vi "FPGA_Check_Pins_host.vi"() -> ()   [LabVIEW 2018]
uses:
  <vilib>/userdefined/High Color/nirio_resource_hc.ctl
  <vilib>/FPGAPlugInAG/PXI-7951R/niLvFpga_Open_PXI-7951R.vi
  <vilib>/rvi/interface/common/dynamic/niFpgaDynamicAddResources.vi
  <vilib>/FPGAPlugInAG/Dynamic/niLvFpga_Reset_Dynamic.vi
  <vilib>/FPGAPlugInAG/Dynamic/niLvFpga_Run_Dynamic.vi
  <vilib>/Utility/error.llb/Error Cluster From Error Code.vi
  <vilib>/rvi/errors/niLvFpgaAdjustHostInterfaceError.vi
  <vilib>/FPGAPlugInAG/Dynamic/niLvFpga_Close_Dynamic.vi
  <vilib>/rvi/interface/nirviOpenFPGA/nirviOpenFPGA.xnode
  FPGA Bitfiles/FPGACheckPins_FPGATarget_FPGACheckPinstar_o4gGUkoAHio.lvbitx
  <vilib>/rvi/interface/nirviMethod/nirviMethod.xnode
  <vilib>/rvi/interface/nirviReadWriteControl/nirviReadWriteControl.xnode
  <vilib>/rvi/interface/nirviCloseFPGA/nirviCloseFPGA.xnode
  <vilib>/rvi/interface/Simulation/niFpgaSimulationCallBeginRW.vi
  NiFpgaLv.dll
panel:
  in  "Tab Control":enum32{"Main", "Service"}(tab)
  out "output array":bool[][](array[boolean])
  out "appended array":bool[](array[boolean])
  out "Ток, А":dbl(knob) scale=0.0..1.0
  in  "FPGA slot name":T1="PXI1Slot2" caption="RIO Device"
  out "error out (4110)":errorcluster
  out "error out FPGA":errorcluster
  in  "Power Resource":refnum<k15>="PXI1Slot3"
  in  "Output enabled CH1":bool
  in  "Stop Program":bool
  in  "Write to Read":bool
  out "Read B":u32=117440511 format="%b"
  out "Read A":u32=134217727 format="%b"
  out "WRITE TOTAL":u32=38686286 format="%b"
  in  "Ток, А  2":dbl=0.9 caption="Current limit CH1" format="%#_13g"
  in  "Напряжение, В":dbl=3.0
  out "U CH0.1, В":dbl=0.000596728952024882
  out "I CH0.1, A":dbl=2.324707150327661e-06
  in  "Write to PFI 2":u8=6 format="%b"
  in  "Write to PFI":u16(ring)=1 items=["Manual mode", "Random", "Increment", "Chess", "NChess", "Only one", "Zero", "Check one"]
  in  "Cycle":bool=TRUE
  in  "Write to port  2":u8=248 format="%b"
  out "Read PFI 2":i16=1
  out "Read PFI 3":i16=1
  out "Read PFI 1":i16
  out "Чтение PFI 1":i16=1
  out "Чтение PFI 2":i16=1
  out "Чтение PFI 3":i16=1
  out "Read B2":u32=255 format="%b"
  out "Read B1":u32=255 format="%b"
  out "Read B0":u32=255
  out "Read А2":u32=255 format="%b"
  out "Read А1":u32=255 format="%b"
  out "Read А0":u32=255
  in  "Write to port":u16(ring)=1 items=["Manual mode", "Random", "Increment", "Chess", "NChess", "Only one", "Zero", "Chess diagonal", "NChess diagonal"]
  out "Delay B to A, такт":i16
  out "Delay A to B, такт":i16
  # "0          1          2         3          4          5          6          7"
  # "Port 0"
  # "PFI 1"
  # "Port 1"
  # "PFI 2"
  # "Port 2"
  # "PFI 3"
  # "Control"
  # "Чтение портов"
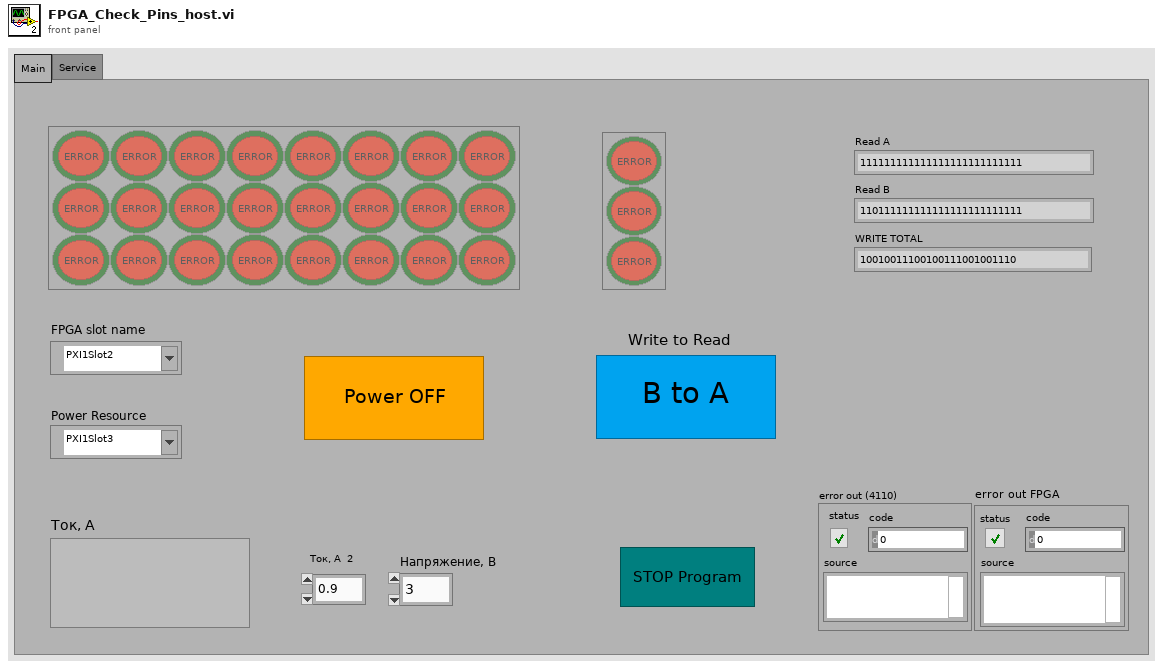
[diagram p1: front panel]
types:
  T1 = typedef "nirio_resource_hc.ctl" = tag
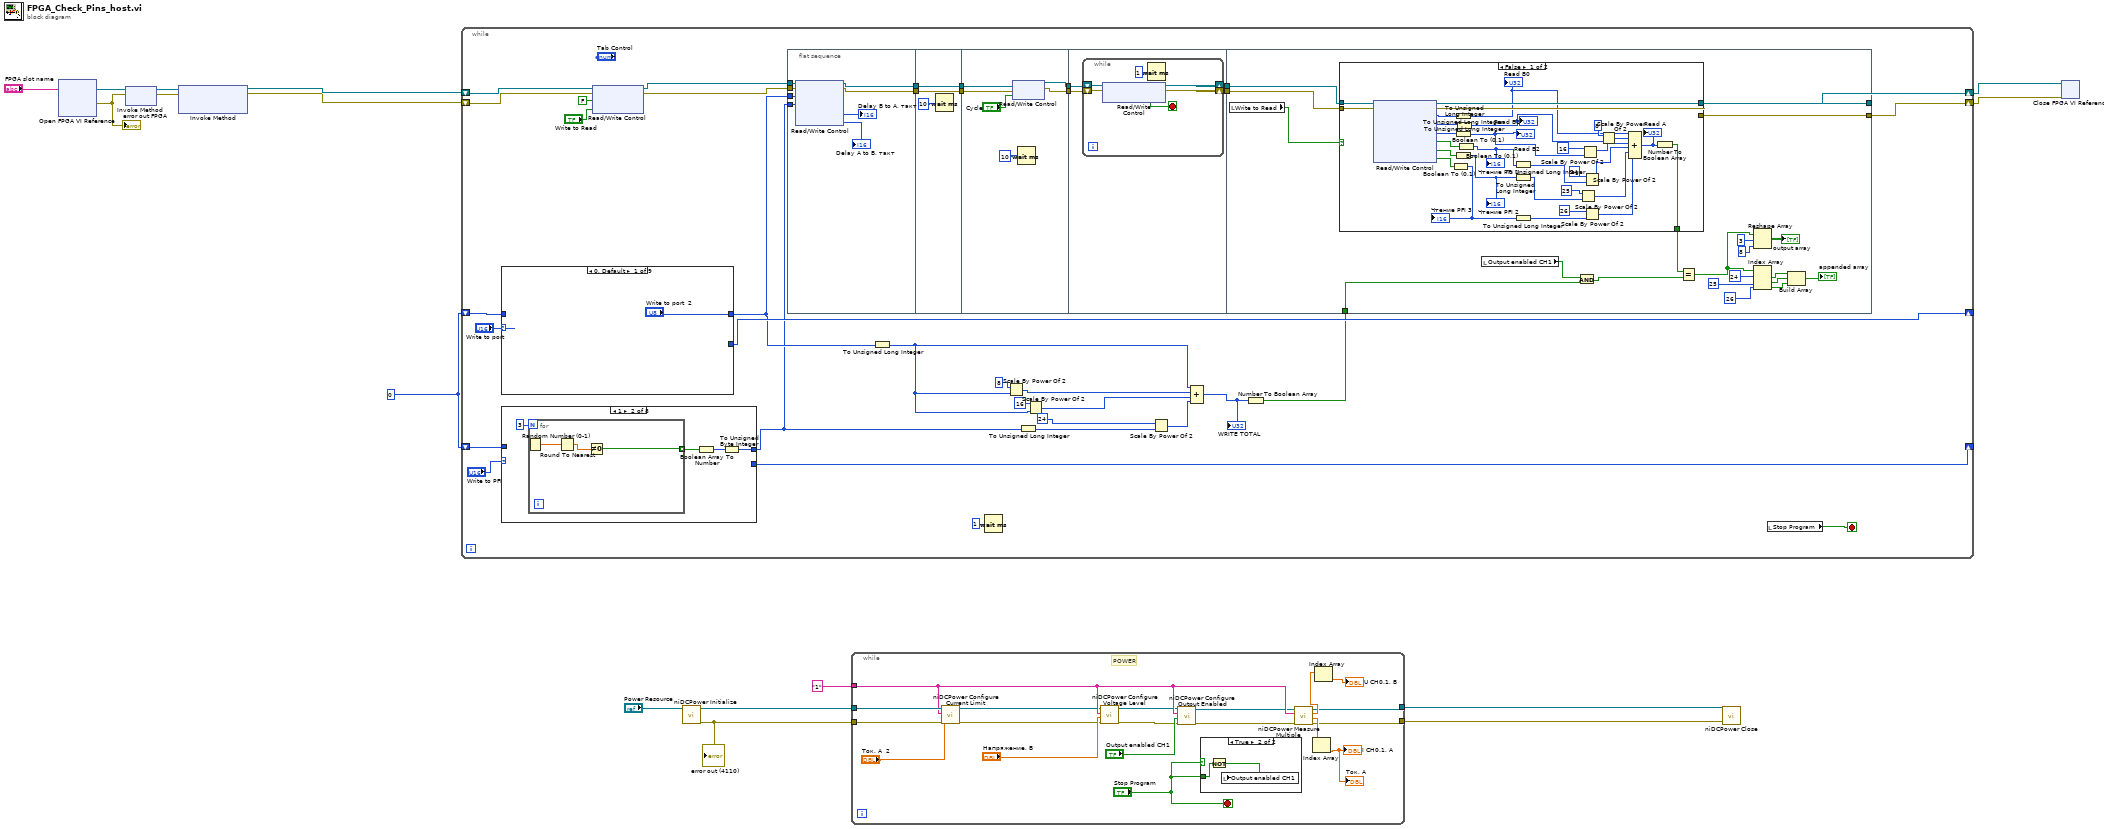
[diagram p0: block diagram]
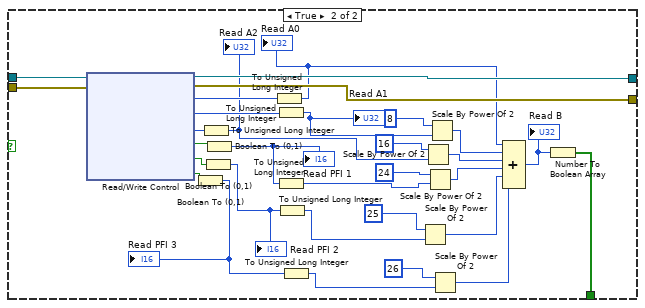
[diagram p2: hidden frame]
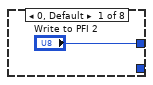
[diagram p3: hidden frame]
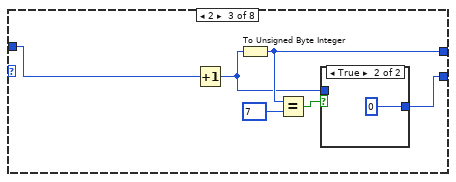
[diagram p4: hidden frame]
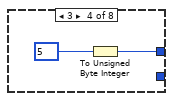
[diagram p6: hidden frame]
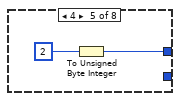
[diagram p7: hidden frame]
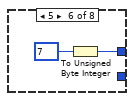
[diagram p8: hidden frame]
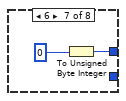
[diagram p9: hidden frame]
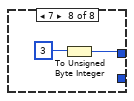
[diagram p10: hidden frame]
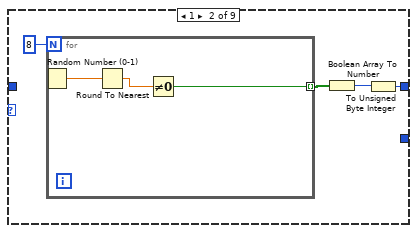
[diagram p11: hidden frame]
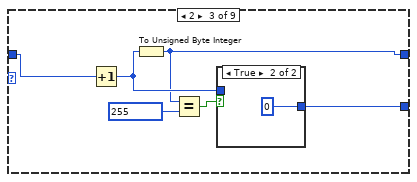
[diagram p12: hidden frame]
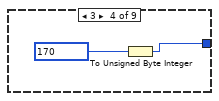
[diagram p14: hidden frame]
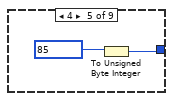
[diagram p15: hidden frame]
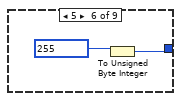
[diagram p16: hidden frame]
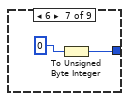
[diagram p17: hidden frame]
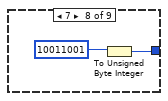
[diagram p18: hidden frame]
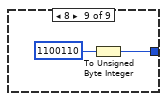
[diagram p19: hidden frame]
diagram:
  w1 = 0
  n1 = xnode "Open FPGA VI Reference"("resource name"="FPGA slot name") -> ("FPGA VI Reference Out"=w9:refnum<k20>, "error out"=w8:errorcluster)  [unwired: 1 in]
  "error out FPGA" <- w8
  n2 = xnode "Invoke Method"("FPGA VI Reference In"=w9, "error in"=w8) -> ("FPGA VI Reference Out"=w7:refnum<k20>, "error out"=w6:errorcluster)
  n3 = xnode ("Invoke Method")("FPGA VI Reference In"=w7, "error in"=w6) -> ("FPGA VI Reference Out"=w3:refnum<k20>, "error out"=w2:errorcluster)  [unwired: 1 in]
  n4 = while {
    shift-right: [w19] -> w5
    shift-left: w3 -> [w37]
    shift-right: [w18] -> w4
    shift-left: w2 -> [w36]
    shift-right: [w40] -> _
    shift-left: w1 -> [w41]
    shift-right: [w38] -> _
    shift-left: w1 -> [w39]
    stop <- w22 stop-if-true
    n5 = case shown="0, Default" "Write to port" {
      tunnel: ["Write to port  2" w189 w197 w204 w207 w209 w211 w213 w214] -> w33
      tunnel: w39 -> [_ _ w198 _ _ _ _ _ _]
      tunnel: [_ _ w196 _ _ _ _ _ _] -> w38
      frame 0, Default {
      }
      frame 1 {
        n6 = for {
          N: 8 -> [_]
          tunnel: [w193] -> w191 mode=indexing
          n7 = Random Number (0-1)() -> (number: 0 to 1=w195:dbl)
          n8 = Round To Nearest(number=w195) -> (nearest integer value=w194:dbl)
          n9 = Not Equal To 0?(x=w194) -> (x != 0?=w193:bool)
        }
        n10 = Boolean Array To Number(Boolean array=w191) -> (number=w190:u32)
        n11 = To Unsigned Byte Integer(number=w190) -> (unsigned 8bit integer=w189:u8)
      }
      frame 2 {
        n12 = Increment(x=w198) -> (x+1=w201:i32)
        n13 = To Unsigned Byte Integer(number=w201) -> (unsigned 8bit integer=w197:u8)
        n14 = Equal?(x=w197, y=u8 255) -> (x = y?=w200:bool)
        n15 = case shown="True" w200 {
          tunnel: [w202 0] -> w196
          tunnel: w201 -> [w202 _]
          frame False {
          }
          frame True {
          }
        }
      }
      frame 3 {
        n16 = To Unsigned Byte Integer(number=170) -> (unsigned 8bit integer=w204:u8)
      }
      frame 4 {
        n17 = To Unsigned Byte Integer(number=85) -> (unsigned 8bit integer=w207:u8)
      }
      frame 5 {
        n18 = To Unsigned Byte Integer(number=255) -> (unsigned 8bit integer=w209:u8)
      }
      frame 6 {
        n19 = To Unsigned Byte Integer(number=0) -> (unsigned 8bit integer=w211:u8)
      }
      frame 7 {
        n20 = To Unsigned Byte Integer(number=10011001) -> (unsigned 8bit integer=w213:u8)
      }
      frame 8 {
        n21 = To Unsigned Byte Integer(number=1100110) -> (unsigned 8bit integer=w214:u8)
      }
    }
    n22 = case shown="1" "Write to PFI" {
      tunnel: ["Write to PFI 2" w163 w173 w179 w181 w183 w185 w187] -> w30
      tunnel: w41 -> [_ _ w175 _ _ _ _ _]
      tunnel: [_ _ w171 _ _ _ _ _] -> w40
      frame 0, Default {
      }
      frame 1 {
        n23 = for {
          N: 3 -> [_]
          tunnel: [w167] -> w165 mode=indexing
          n24 = Random Number (0-1)() -> (number: 0 to 1=w169:dbl)
          n25 = Round To Nearest(number=w169) -> (nearest integer value=w168:dbl)
          n26 = Not Equal To 0?(x=w168) -> (x != 0?=w167:bool)
        }
        n27 = Boolean Array To Number(Boolean array=w165) -> (number=w164:u32)
        n28 = To Unsigned Byte Integer(number=w164) -> (unsigned 8bit integer=w163:u8)
      }
      frame 2 {
        n29 = Increment(x=w175) -> (x+1=w170:i32)
        n30 = To Unsigned Byte Integer(number=w170) -> (unsigned 8bit integer=w173:u8)
        n31 = Equal?(x=w173, y=u8 7) -> (x = y?=w172:bool)
        n32 = case shown="True" w172 {
          tunnel: [w176 0] -> w171
          tunnel: w170 -> [w176 _]
          frame False {
          }
          frame True {
          }
        }
      }
      frame 3 {
        n33 = To Unsigned Byte Integer(number=5) -> (unsigned 8bit integer=w179:u8)
      }
      frame 4 {
        n34 = To Unsigned Byte Integer(number=2) -> (unsigned 8bit integer=w181:u8)
      }
      frame 5 {
        n35 = To Unsigned Byte Integer(number=7) -> (unsigned 8bit integer=w183:u8)
      }
      frame 6 {
        n36 = To Unsigned Byte Integer(number=0) -> (unsigned 8bit integer=w185:u8)
      }
      frame 7 {
        n37 = To Unsigned Byte Integer(number=3) -> (unsigned 8bit integer=w187:u8)
      }
    }
    n38 = xnode "Read/Write Control"("FPGA VI Reference In"=w37, "error in"=w36, "Cycle"=FALSE, "A to B/B to A"="Write to Read") -> ("FPGA VI Reference Out"=w35:refnum<k20>, "error out"=w34:errorcluster)
    n39 = flat-sequence {
      tunnel: w35 -> [w58]
      tunnel: w34 -> [w57]
      tunnel: w33 -> [w56]
      tunnel: w30 -> [w55]
      tunnel: [w60] -> w29
      tunnel: [w59] -> w28
      tunnel: w29 -> [w63]
      tunnel: w28 -> [w62]
      tunnel: [w63] -> w27
      tunnel: [w62] -> w26
      tunnel: w27 -> [w69]
      tunnel: w26 -> [w68]
      tunnel: [w67] -> w25
      tunnel: [w66] -> w24
      tunnel: w25 -> [w71]
      tunnel: w24 -> [w70]
      tunnel: [w73] -> w21
      tunnel: [w72] -> w20
      tunnel: w21 -> [w98]
      tunnel: w20 -> [w97]
      tunnel: [w96] -> w19
      tunnel: [w95] -> w18
      tunnel: w17 -> [w94]
      frame #0 {
        n40 = xnode "Read/Write Control"("FPGA VI Reference In"=w58, "error in"=w57, "Write to"=w56, "Write to PFI"=w55) -> ("FPGA VI Reference Out"=w60:refnum<k20>, "error out"=w59:errorcluster, "Delay B to A"=→"Delay B to A, такт":i16, "Delay A to B"=→"Delay A to B, такт":i16)
      }
      frame #1 {
        n41 = Wait (ms)(milliseconds to wait=u32 10) -> ()  [unwired: 1 out]
      }
      frame #2 {
        n42 = xnode "Read/Write Control"("FPGA VI Reference In"=w69, "error in"=w68, "Cycle"="Cycle") -> ("FPGA VI Reference Out"=w67:refnum<k20>, "error out"=w66:errorcluster)
        n43 = Wait (ms)(milliseconds to wait=u32 10) -> ()  [unwired: 1 out]
      }
      frame #3 {
        n44 = while {
          shift-right: [w79] -> w73
          shift-left: w71 -> [w77]
          shift-right: [w78] -> w72
          shift-left: w70 -> [w76]
          stop <- w74 stop-if-true
          n45 = xnode "Read/Write Control"("FPGA VI Reference In"=w77, "error in"=w76) -> ("FPGA VI Reference Out"=w79:refnum<k20>, "error out"=w78:errorcluster, "Operation compl"=w74:bool)
          n46 = Wait (ms)(milliseconds to wait=u32 1) -> ()  [unwired: 1 out]
        }
      }
      frame #4 {
        n47 = local read "Write to Read"() -> (w99:bool)
        n48 = case shown="False" w99 {
          tunnel: [w130 w161] -> w96
          tunnel: [w129 w160] -> w95
          tunnel: [w118 w155] -> w91
          tunnel: w98 -> [w101 w132]
          tunnel: w97 -> [w100 w131]
          frame False {
            n49 = xnode "Read/Write Control"("FPGA VI Reference In"=w101, "error in"=w100) -> ("FPGA VI Reference Out"=w130:refnum<k20>, "error out"=w129:errorcluster, "Read Port 0 A"=w124:u8, "Read Port 1 A"=w123:u8, "Read Port 2 A"=w122:u8, "DDCA_PFI1_Read"=w114:bool, "DDCA_PFI2_Read"=w112:bool, "DDCA_PFI3_Read"=w113:bool)
            n50 = Boolean To (0,1)(Boolean=w113) -> (0, 1=w105:i16)
            "Чтение PFI 3" <- w105
            n51 = To Unsigned Long Integer(number=w122) -> (unsigned 32bit integer=w121:u32)
            "Read B2" <- w121
            n52 = To Unsigned Long Integer(number=w124) -> (unsigned 32bit integer=w119:u32)
            "Read B0" <- w119
            n53 = Boolean To (0,1)(Boolean=w112) -> (0, 1=w106:i16)
            "Чтение PFI 2" <- w106
            n54 = To Unsigned Long Integer(number=w123) -> (unsigned 32bit integer=w120:u32)
            "Read B1" <- w120
            n55 = Boolean To (0,1)(Boolean=w114) -> (0, 1=w107:i16)
            "Чтение PFI 1" <- w107
            n56 = To Unsigned Long Integer(number=w107) -> (unsigned 32bit integer=w102:u32)
            n57 = To Unsigned Long Integer(number=w106) -> (unsigned 32bit integer=w103:u32)
            n58 = To Unsigned Long Integer(number=w105) -> (unsigned 32bit integer=w104:u32)
            n59 = Scale By Power Of 2(n=i16 25, x=w103) -> (x*2^n=w111:u32)
            n60 = Scale By Power Of 2(n=i16 16, x=w121) -> (x*2^n=w117:u32)
            n61 = Scale By Power Of 2(n=i16 24, x=w102) -> (x*2^n=w116:u32)
            n62 = Scale By Power Of 2(n=i16 26, x=w104) -> (x*2^n=w110:u32)
            n63 = Scale By Power Of 2(n=i16 8, x=w120) -> (x*2^n=w127:u32)
            n64 = Compound Arithmetic op=unknown(w119, w127, w117, w116, w111, w110) -> (w128:u32)
            "Read A" <- w128
            n65 = Number To Boolean Array(number=w128) -> (Boolean array=w118:bool[])
          }
          frame True {
            n66 = xnode ("Read/Write Control")("FPGA VI Reference In"=w132, "error in"=w131) -> ("FPGA VI Reference Out"=w161:refnum<k20>, "error out"=w160:errorcluster, "Read Port 0 B"=w154:u8, "Read Port 1 B"=w151:u8, "Read Port 2 B"=w150:u8, "DDCB_PFI1_Read"=w144:bool, "DDCB_PFI2_Read"=w145:bool, "DDCB_PFI3_Read"=w146:bool)
            n67 = Boolean To (0,1)(Boolean=w146) -> (0, 1=w138:i16)
            "Read PFI 3" <- w138
            n68 = To Unsigned Long Integer(number=w150) -> (unsigned 32bit integer=w149:u32)
            "Read А2" <- w149
            n69 = Boolean To (0,1)(Boolean=w145) -> (0, 1=w135:i16)
            "Read PFI 2" <- w135
            n70 = Boolean To (0,1)(Boolean=w144) -> (0, 1=w134:i16)
            "Read PFI 1" <- w134
            n71 = To Unsigned Long Integer(number=w154) -> (unsigned 32bit integer=w153:u32)
            "Read А0" <- w153
            n72 = To Unsigned Long Integer(number=w151) -> (unsigned 32bit integer=w152:u32)
            "Read А1" <- w152
            n73 = To Unsigned Long Integer(number=w134) -> (unsigned 32bit integer=w133:u32)
            n74 = To Unsigned Long Integer(number=w135) -> (unsigned 32bit integer=w136:u32)
            n75 = To Unsigned Long Integer(number=w138) -> (unsigned 32bit integer=w137:u32)
            n76 = Scale By Power Of 2(n=i16 25, x=w136) -> (x*2^n=w142:u32)
            n77 = Scale By Power Of 2(n=i16 16, x=w149) -> (x*2^n=w158:u32)
            n78 = Scale By Power Of 2(n=24, x=w133) -> (x*2^n=w143:u32)
            n79 = Scale By Power Of 2(n=i16 8, x=w152) -> (x*2^n=w159:u32)
            n80 = Scale By Power Of 2(n=i16 26, x=w137) -> (x*2^n=w141:u32)
            n81 = Compound Arithmetic op=ADD(w153, w159, w158, w143, w142, w141) -> (w156:u32)
            "Read B" <- w156
            n82 = Number To Boolean Array(number=w156) -> (Boolean array=w155:bool[])
          }
        }
        n83 = local read "Output enabled CH1"() -> (w93:bool)
        n84 = And(x=w93, y=w94) -> (x .and. y?=w92:bool[])
        n85 = Equal?(x=w91, y=w92) -> (x = y?=w85:bool[])
        n86 = Index Array(array=w85, index #1=24 ("index"), index #2=25 ("index"), index #3=26 ("index")) -> (element #1=w87:bool, element #2=w88:bool, element #3=w89:bool)
        n87 = Reshape Array(w85, 3 ("dimension size"), 8 ("dimension size")) -> (→"output array":bool[][])
        n88 = Build Array(w87, w88, w89) -> (→"appended array":bool[])
      }
    }
    n89 = To Unsigned Long Integer(number=w33) -> (unsigned 32bit integer=w47:u32)
    n90 = Wait (ms)(milliseconds to wait=u32 1) -> ()  [unwired: 1 out]
    n91 = Scale By Power Of 2(n=i16 8, x=w47) -> (x*2^n=w51:u32)
    n92 = To Unsigned Long Integer(number=w30) -> (unsigned 32bit integer=w46:u32)
    n93 = Scale By Power Of 2(n=i16 16, x=w47) -> (x*2^n=w52:u32)
    n94 = Scale By Power Of 2(n=i16 24, x=w46) -> (x*2^n=w44:u32)
    n95 = Compound Arithmetic op=ADD(w47, w51, w52, w44) -> (w50:u32)
    "WRITE TOTAL" <- w50
    n96 = Number To Boolean Array(number=w50) -> (Boolean array=w17:bool[])
    n97 = local read "Stop Program"() -> (w22:bool)
  }
  n98 = call <instrlib>:"niDCPower Initialize.vi"("resource name"="Power Resource") -> ("error out"=w15:errorcluster, "instrument handle out"=w14:refnum<k15>)  [unwired: 3 in, 6 out]
  "error out (4110)" <- w15
  n99 = while {
    tunnel: [w222] -> w12
    tunnel: [w221] -> w13
    tunnel: "1" ("Channel name") -> [w227]
    tunnel: w15 -> [w228]
    tunnel: w14 -> [w229]
    stop <- "Stop Program" stop-if-true
    # "POWER"
    n100 = call <instrlib>:"niDCPower Configure Current Limit.vi"("error in (no error)"=w228, "current limit"="Ток, А  2", "channel name"=w227, "instrument handle"=w229) -> ("error out"=w226:errorcluster, "instrument handle out"=w225:refnum<k15>)  [unwired: 6 in]
    n101 = call <instrlib>:"niDCPower Configure Voltage Level.vi"("error in (no error)"=w226, "voltage level"="Напряжение, В", "channel name"=w227, "instrument handle"=w225) -> ("error out"=w223:errorcluster, "instrument handle out"=w224:refnum<k15>)  [unwired: 6 in]
    n102 = call <instrlib>:"niDCPower Configure Output Enabled.vi"("error in (no error)"=w223, "output enabled"="Output enabled CH1", "channel name"=w227, "instrument handle"=w224) -> ("error out"=w219:errorcluster, "instrument handle out"=w220:refnum<k15>)  [unwired: 6 in]
    n103 = case shown="True" "Stop Program" {
      tunnel: "Stop Program" -> [_ w236]
      frame False {
      }
      frame True {
        n104 = Not(x=w236) -> (.not. x?=w235:bool)
        n105 = local write "Output enabled CH1"(w235) -> ()
      }
    }
    n106 = call <instrlib>:"niDCPower Measure Multiple.vi"("error in (no error)"=w219, "channel name"=w227, "instrument handle"=w220) -> ("error out"=w222:errorcluster, "current measurements"=w233:dbl[], "voltage measurements"=w231:dbl[], "instrument handle out"=w221:refnum<k15>)  [unwired: 5 in]
    n107 = Index Array(array=w233) -> (element=→"I CH0.1, A" →"Ток, А":dbl)  [unwired: 1 in]
    n108 = Index Array(array=w231) -> (element=→"U CH0.1, В":dbl)  [unwired: 1 in]
  }
  n109 = call <instrlib>:"niDCPower Close.vi"("error in (no error)"=w12, "instrument handle"=w13) -> ()  [unwired: 9 in, 1 out]
  n110 = xnode "Close FPGA VI Reference"("FPGA VI Reference In"=w5, "error in"=w4) -> ()  [unwired: 1 out]
